vi "Stop.vi"(8 "error in (no error)":errorcluster, 11 "Scope PXI in":refnum<class "Scope PXI.lvclass">) -> (0 "error out":errorcluster, 3 "Scope PXI out":refnum<class "Scope PXI.lvclass">)   [LabVIEW 2023, in "Scope.lvlib" / "Scope PXI.lvlib" / "Scope PXI.lvclass"]
uses:
  Scope PXI.lvclass
  Scope PXI.lvclass/Scope PXI.ctl
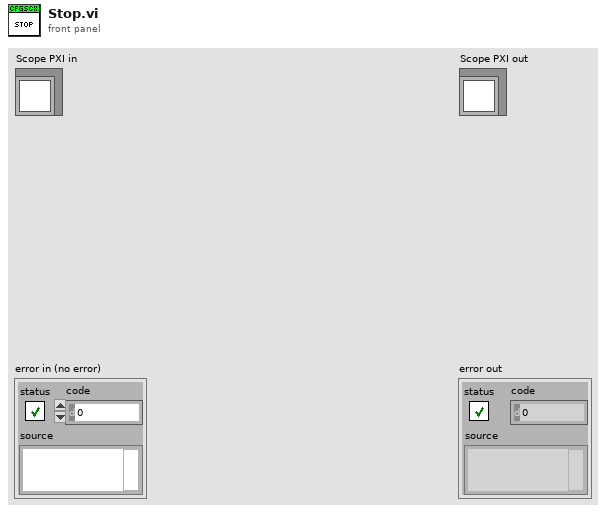
[diagram p1: front panel]
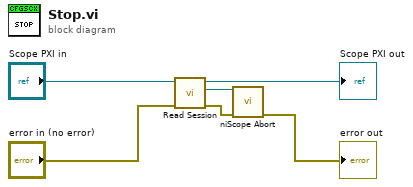
[diagram p0: block diagram]
diagram:
  n1 = call "Read Session.vi"("error in (no error)"="error in (no error)", "Scope PXI in"="Scope PXI in") -> ("error out"=w1:errorcluster, "session"=w4:refnum<k15>, "Scope PXI out"=→"Scope PXI out":refnum<class "Scope PXI.lvclass">)  [unwired: 7 in]
  n2 = call <instrlib>:"niScope Abort.vi"("instrument handle"=w4, "error in"=w1) -> ("error out"=→"error out":errorcluster)  [unwired: 12 in, 1 out]
